vi "Get Number of Points Completed.vi"(8 "error in":errorcluster, 11 "eye scan in":refnum<class "niHighSpeedSerial Eye Scan v1 Host.lvclass">) -> (0 "error out":errorcluster, 2 "number of points completed":i32, 3 "eye scan out":refnum<class "niHighSpeedSerial Eye Scan v1 Host.lvclass">)   [LabVIEW 2014, in "niHighSpeedSerial Eye Scan v1 Host.lvclass"]
doc: "Returns the number of points completed.\n\n<B>Input Parameters</B>\n\n<B>error in</B> describes error conditions that occur before this node runs. This input provides standard 'error in' functionality.\n\n<B>eye scan in</B> Takes in a reference to your session from the previous VI.\n\n<B>Output Parameters</B>\n\n<B>error out</B> contains error information. This output provides standard 'error out' functionality.\n\n<B>number of points completed</B> is the number of points which have been completed since Eye Scan began measuring.\n\n<B>eye scan out</B> passes a reference to your session to the next VI."
uses:
  <instrlib>/niHighSpeedSerial/Eye Scan/v1/Host/Eye Scan/niHighSpeedSerial Eye Scan v1 Host.lvclass
  <instrlib>/niHighSpeedSerial/Eye Scan/v1/Host/Eye Scan/niHighSpeedSerial Eye Scan v1 Host.lvclass/niHighSpeedSerial Eye Scan v1 Host.ctl
  <vilib>/Utility/error.llb/Error Cluster From Error Code.vi
  <vilib>/ErrorRing/Error Ring.xnode
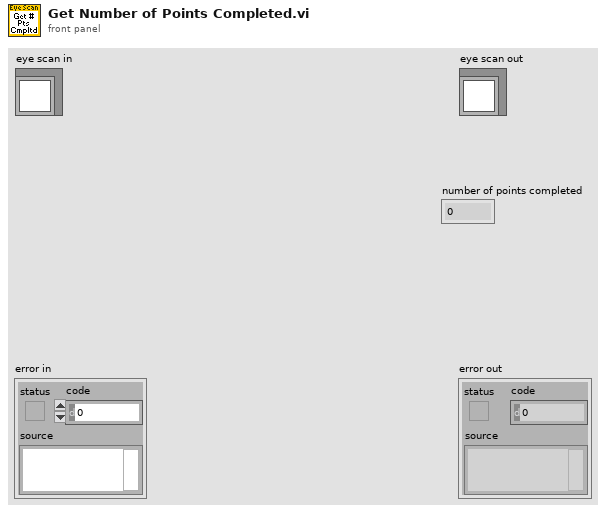
[diagram p1: front panel]
types:
  T1 = typedef "niHighSpeedSerial Eye Scan v1 Host.lvclass/Private Data.ctl" = cluster{"instruction target":refnum<class "niInstr Instruction Target v1 Host.lvclass">, "channels":T2[], "measure state":T3, "rx output divider":T4, "equalization mode":T5, "rx data width":T6, "BER floor":dbl, "number of points completed":i32, "rx output divider configured?":bool, "equalization mode configured?":bool, "rx data width configured?":bool}
  T2 = typedef "niHighSpeedSerial Eye Scan v1 Host.lvclass/Channel Data.ctl" = cluster{"instance":u8, "channel":refnum<class "niHighSpeedSerial Eye Scan Single Point v1 Host.lvclass">, "point iterator":refnum<class "niHighSpeedSerial Eye Scan Point Iterator v1 Host.lvclass">}
  T3 = typedef "niHighSpeedSerial Eye Scan v1 Host.lvclass/Measure State.ctl" = enum16{"Uninitialized", "Initialized", "Ready", "Measuring", "Finished", "Aborted"}
  T4 = typedef "niHighSpeedSerial Eye Scan Common v1 Host.lvlib/RX Output Divider.ctl" = enum16{"1", "2", "4", "8", "16"}
  T5 = typedef "niHighSpeedSerial Eye Scan Common v1 Host.lvlib/Equalization Mode.ctl" = enum16{"DFE", "LPM"}
  T6 = typedef "niHighSpeedSerial Eye Scan Common v1 Host.lvlib/Data Width.ctl" = enum16{"16 Bit", "20 Bit", "32 Bit", "40 Bit"}
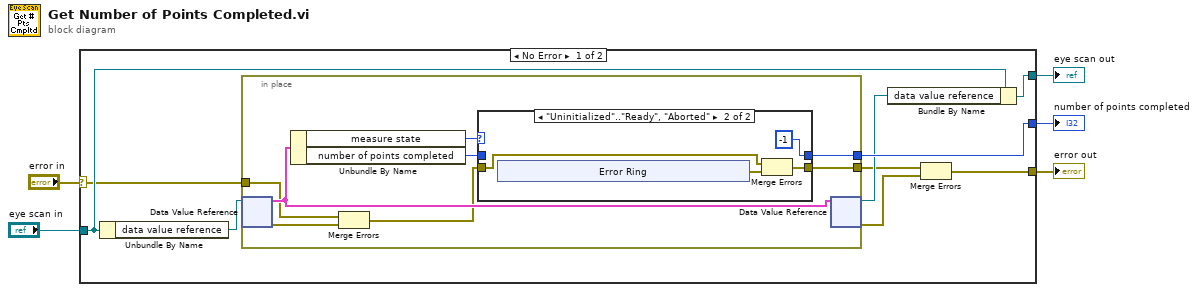
[diagram p0: block diagram]
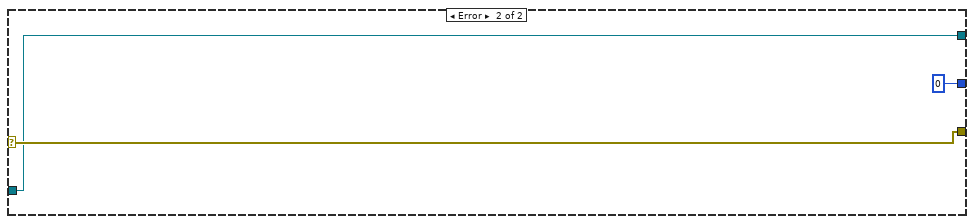
[diagram p3: hidden frame]
diagram:
  n1 = case shown="No Error" "error in" {
    selector: "error in" -> [w7 w35]
    tunnel: [w6 w35] -> w2
    tunnel: [w11 w34] -> w3
    tunnel: "eye scan in" -> [w12 w34]
    tunnel: [w13 0 ("number of points completed")] -> w1
    frame No Error {
      n2 = Unbundle By Name(w12) -> ("data value reference"=w14:refnum<data-value>)
      n3 = in-place {
        in-place-border: [w18] -> w13
        in-place-border: w7 -> [w20]
        in-place-border: [w15] -> w9
        n4 = in-place-dvr #1(w14) -> (w22:T1, w21:errorcluster)
        n5 = Unbundle By Name(w22) -> ("measure state"=w19:T3, "number of points completed"=w17:i32)
        n6 = Merge Errors(w20, w21) -> (w16:errorcluster)
        n7 = case shown="\"Uninitialized\"..\"Ready\", \"Aborted\"" w19 {
          tunnel: [w24 -1 ("number of points completed")] -> w18
          tunnel: w17 -> [w24 _]
          tunnel: w16 -> [w23 w27]
          tunnel: [w23 w26] -> w15
          frame "Measuring", "Finished" {
          }
          frame "Uninitialized".."Ready", "Aborted" {
            n8 = xnode "Error Ring"() -> ("error out"=w25:errorcluster)
            n9 = Merge Errors(w27, w25) -> (w26:errorcluster)
          }
        }
        n10 = in-place-dvr #1(w22) -> (w10:refnum<data-value>, w8:errorcluster)
      }
      n11 = Bundle By Name(cluster=w12, "data value reference"=w10) -> (w11:refnum<class "niHighSpeedSerial Eye Scan v1 Host.lvclass">)
      n12 = Merge Errors(w9, w8) -> (w6:errorcluster)
    }
    frame Error {
    }
  }
  "error out" <- w2
  "eye scan out" <- w3
  "number of points completed" <- w1
